vi "Get Windows File Locations.vi"(8 "error in (no error)":errorcluster, 11 "Requested Path":i32(ring) items=["Desktop"=0, "Personal Documents"=5, "AppData"=26, "Local AppData"=28, "Common AppData"=35, "Program Files"=38, "Program Files Common"=43, "Common Documents"=46]) -> (0 "error out":errorcluster, 3 "path":path)   [LabVIEW 2017]
uses:
  shell32.dll
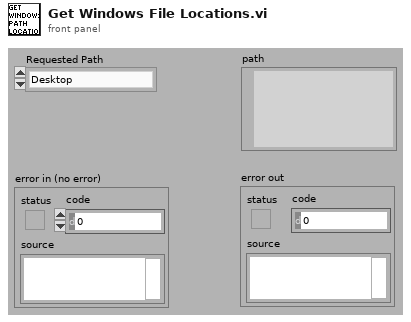
[diagram p1: front panel]
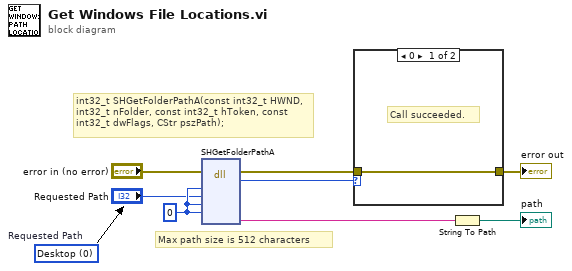
[diagram p0: block diagram]
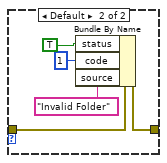
[diagram p2: hidden frame]
diagram:
  (unwired) 0 items=["Desktop"=0, "Personal Documents"=5, "AppData"=26, "Local AppData"=28, "Common AppData"=35, "Program Files"=38, "Program Files Common"=43, "Common Documents"=46]  # Requested Path
  w5 = 0 ("HWND")
  # "int32_t SHGetFolderPathA(const int32_t HWND, int32_t nFolder, const int32_t hToken, const int32_t dwFlags, CStr pszPath);"
  # "Max path size is 512 characters"
  n1 = dll-call lib="shell32.dll" fn="SHGetFolderPathA"(error in="error in (no error)", "HWND"=w5, "nFolder"="Requested Path", "hToken"=w5, "dwFlags"=w5) -> (error out=w3:errorcluster, "Succeeded"=w4:i32, "pszPath"=w7:string)  [unwired: 7 in, 1 out]
  n2 = case shown="0" w4 {
    tunnel: w3 -> [w9 w14]
    tunnel: [w9 w10] -> w2
    frame 0 {
      # "Call succeeded."
    }
    frame Default {
      n3 = Bundle By Name(cluster=w14, "status"=TRUE, "code"=1, "source"="Invalid Folder") -> (w10:errorcluster)
    }
  }
  "error out" <- w2
  n4 = String To Path(string=w7) -> (path=→"path":path)
